vi "Set Chamber.vi"(8 "error in (no error)":errorcluster, 10 "Action":T1="Seal", 11 "instrument.PPMS":refnum<class "instrument.PPMS.lvclass">) -> (0 "error out":errorcluster, 3 "instrument.PPMS out":refnum<class "instrument.PPMS.lvclass">)   [LabVIEW 2019, in "instrument.PPMS.lvclass"]
uses:
  instrument.PPMS.lvclass
  C:/Program Files (x86)/National Instruments/LabVIEW 2019/user.lib/LevyLab/Instrument Framework/SMOs/Instrument/Instrument.lvclass
  Typedefs/PPMS.Chamber Command--enum.ctl
  Typedefs/PPMS.Commands-enum.ctl
  <userlib>/LevyLab/Instrument Framework/SMOs/Instrument/Instrument.lvclass/Instrument.ctl
  b51c84d0-5fd0-4aec-a8e9-50ff2b5b00c7.vi
  <vilib>/AdvancedString/1D String Array to Delimited String.vi
  b51c84d0-5fd0-4aec-a8e9-50ff2b5b00c7.vi/da421d9b-e94e-4cca-bf5b-f9d20a599c0f.vi
  b51c84d0-5fd0-4aec-a8e9-50ff2b5b00c7.vi/da421d9b-e94e-4cca-bf5b-f9d20a599c0f.vi/3fe1bbbf-522b-4775-b886-4d394b683356.vi
  <userlib>/LevyLab/Instrument Framework/SMOs/Instrument/API/Send and Receive.vi
  b51c84d0-5fd0-4aec-a8e9-50ff2b5b00c7.vi/da421d9b-e94e-4cca-bf5b-f9d20a599c0f.vi/610a6a41-d58a-4313-ba82-cae0622802c3.vi
  <userlib>/LevyLab/Instrument Framework/SMOs/Instrument/Private/Get Client Type.vi
  b51c84d0-5fd0-4aec-a8e9-50ff2b5b00c7.vi/da421d9b-e94e-4cca-bf5b-f9d20a599c0f.vi/3fe1bbbf-522b-4775-b886-4d394b683356.vi/c4bf066d-51a2-45c7-9af5-d17cac818fbb.vi
  b51c84d0-5fd0-4aec-a8e9-50ff2b5b00c7.vi/da421d9b-e94e-4cca-bf5b-f9d20a599c0f.vi/3fe1bbbf-522b-4775-b886-4d394b683356.vi/f9d1dcb5-d66b-40ec-a33c-f887ac888bf6.vi
  b51c84d0-5fd0-4aec-a8e9-50ff2b5b00c7.vi/da421d9b-e94e-4cca-bf5b-f9d20a599c0f.vi/610a6a41-d58a-4313-ba82-cae0622802c3.vi/d1819ac0-aa3b-4df9-9960-0218ac92fe2c.vi
  b51c84d0-5fd0-4aec-a8e9-50ff2b5b00c7.vi/da421d9b-e94e-4cca-bf5b-f9d20a599c0f.vi/610a6a41-d58a-4313-ba82-cae0622802c3.vi/462e1cd3-963c-4b9a-9c51-c471ec9c7dab.vi
  b51c84d0-5fd0-4aec-a8e9-50ff2b5b00c7.vi/da421d9b-e94e-4cca-bf5b-f9d20a599c0f.vi/610a6a41-d58a-4313-ba82-cae0622802c3.vi/d1819ac0-aa3b-4df9-9960-0218ac92fe2c.vi/24a41805-8b02-484a-903f-c8578204d8b9.vi
  b51c84d0-5fd0-4aec-a8e9-50ff2b5b00c7.vi/da421d9b-e94e-4cca-bf5b-f9d20a599c0f.vi/610a6a41-d58a-4313-ba82-cae0622802c3.vi/d1819ac0-aa3b-4df9-9960-0218ac92fe2c.vi/e835d68b-3f2c-4479-af9f-b01491fc6e1d.vi
  <userlib>/LevyLab/Instrument Framework/SMOs/Instrument/API/Enum to String.vi
  <userlib>/LevyLab/Instrument Framework/SMOs/Instrument/Private/Get RC Connection Status.vi
  <userlib>/LevyLab/Instrument Framework/SMOs/RemoteControl/API/Send and Receive.vi
  <vilib>/Utility/Data Type/Get Type Information.vi
  <vilib>/JDP Science/JSONtext/JSON text to Variant.vi
  <userlib>/LevyLab/Instrument Framework/SMOs/Instrument/API/Instrument.GetPublicEvents.vi
  <vilib>/JDP Science/JSONtext/Variant to JSON Text.vi
  <vilib>/National Instruments/GUID Generator/Guid Generator.vi
  <userlib>/LevyLab/Instrument Framework/SMOs/Instrument/API/Instrument.MessageToProcess.vi
  <userlib>/LevyLab/Instrument Framework/SMOs/Instrument/Private/Instrument.MessageFromProcess.EventStructure.vi
  <vilib>/Utility/error.llb/Error Cluster From Error Code.vi
  <vilib>/JDP Science/JSONtext/LVClass Serializer/JSONtext LVClass Serializer.lvclass
  <userlib>/LevyLab/Instrument Framework/Instrument Types/Cryostat/Instrument.Cryostat.lvclass
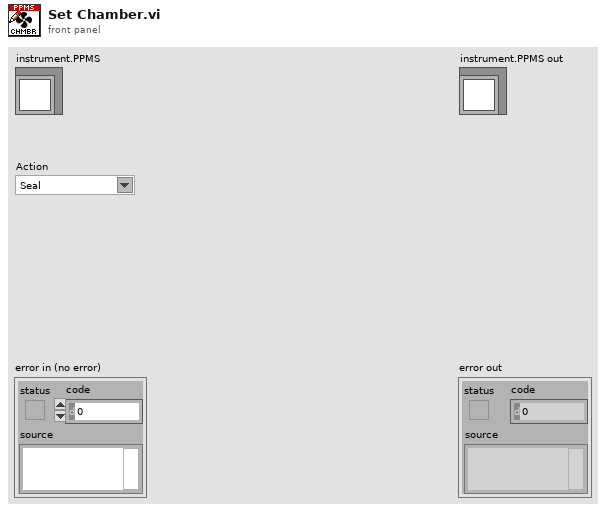
[diagram p1: front panel]
types:
  T1 = typedef "instrument.PPMS.lvclass/PPMS.Chamber Command--enum.ctl" = string
  T2 = typedef "instrument.PPMS.lvclass/PPMS.Commands-enum.ctl" = enum16{"Get Angle", "Get Helium Level", "Get Magnet", "Get Temperature", "Set Angle", "Set Chamber", "Set Magnet", "Set Temperature", "getAll"}
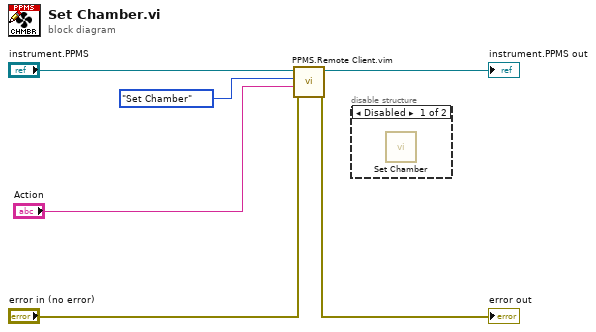
[diagram p0: block diagram]
diagram:
  n1 = call "PPMS.Remote Client.vim"("error in (no error)"="error in (no error)", "params"="Action", "Command"=PPMS.Commands-enum."Set Chamber", "instrument.PPMS in"="instrument.PPMS") -> ("error out"=→"error out":errorcluster, "instrument.PPMS out"=→"instrument.PPMS out":refnum<class "instrument.PPMS.lvclass">)  [unwired: 5 in, 1 out]
  n2 = disable-structure shown="Disabled" {
    frame Disabled {
      n3 = call-parent "Set Chamber.vi"() -> ()  [unwired: 10 in, 2 out]
    }
    frame Enabled {
    }
  }
